vi "Compare and Append Cell.vi"(8 "Schedule Cell B in":refnum<class "Schedule Cell.lvclass">, 11 "Schedule Cell A in":refnum<class "Schedule Cell.lvclass">) -> (0 "Schedule Cell B out":refnum<class "Schedule Cell.lvclass">, 2 "Cell Updated":bool, 3 "Schedule Cell A out":refnum<class "Schedule Cell.lvclass">)   [LabVIEW 2020, in "Run Utilities.lvlib" / "Schedule Cell.lvclass"]
doc: "Compare two cells. If they have the same script the function modifies the cell A accordingly. Otherwise, the function returns unmodified cells."
uses:
  Schedule Cell.lvclass
  Schedule Cell.lvclass/Schedule Cell.ctl
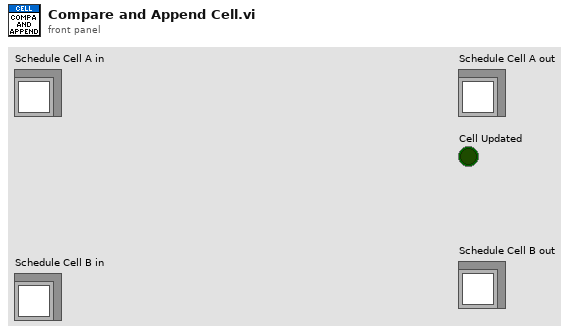
[diagram p1: front panel]
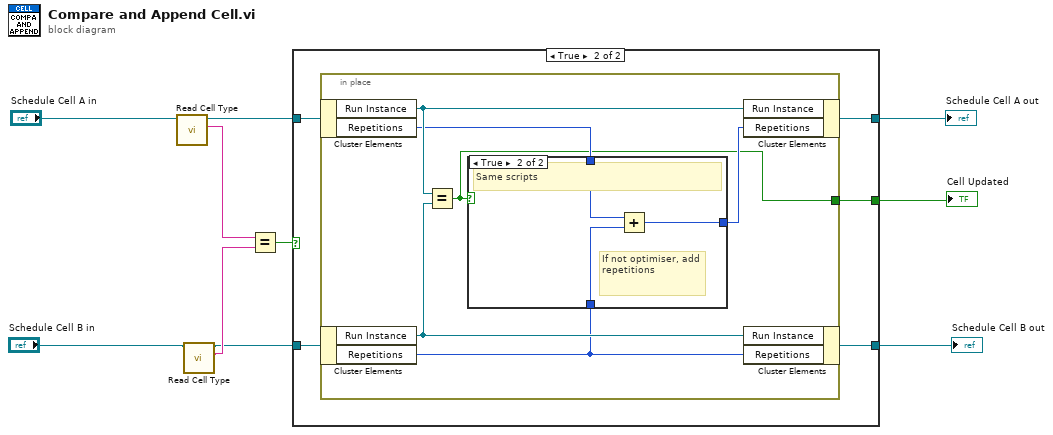
[diagram p0: block diagram]
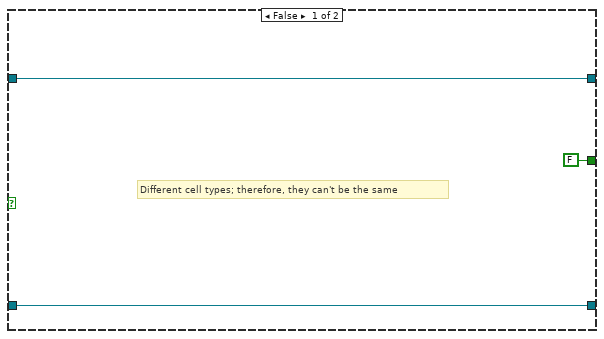
[diagram p2: hidden frame]
diagram:
  n1 = call-dynamic "Read Cell Type.vi"("Schedule Cell in"="Schedule Cell A in") -> ("Cell Type"=w3:string, "Schedule Cell out"=w4:refnum<class "Schedule Cell.lvclass">)  [unwired: 8 in, 1 out]
  n2 = call-dynamic "Read Cell Type.vi"("Schedule Cell in"="Schedule Cell B in") -> ("Cell Type"=w7:string, "Schedule Cell out"=w6:refnum<class "Schedule Cell.lvclass">)  [unwired: 8 in, 1 out]
  n3 = Equal?(x=w3, y=w7) -> (x = y?=w8:bool)
  n4 = case shown="True" w8 {
    tunnel: w4 -> [w12 w18]
    tunnel: [w12 w17] -> w1
    tunnel: [FALSE w16] -> w10
    tunnel: w6 -> [w13 w15]
    tunnel: [w13 w14] -> w9
    frame False {
      # "Different cell types; therefore, they can't be the same"
    }
    frame True {
      n5 = in-place {
        in-place-border: [w19] -> w16
        n6 = in-place-cluster #1(w18) -> ("Run Instance"=w23:refnum<class "Run Instance.lvclass">, "Repetitions"=w21:u32)
        n7 = in-place-cluster #2(w15) -> ("Run Instance"=w24:refnum<class "Run Instance.lvclass">, "Repetitions"=w22:u32)
        n8 = Equal?(x=w23, y=w24) -> (x = y?=w19:bool)
        n9 = case shown="True" w19 {
          tunnel: w22 -> [_ w28]
          tunnel: w21 -> [w25 w27]
          tunnel: [w25 w26] -> w20
          frame False {
            # "Different run cells, do nothing more"
          }
          frame True {
            # "If not optimiser, add repetitions"
            # "Same scripts"
            n10 = Add(x=w27, y=w28) -> (x+y=w26:u32)
          }
        }
        n11 = in-place-cluster #1("Run Instance"=w23, "Repetitions"=w20) -> (w17:refnum<class "Schedule Cell.lvclass">)
        n12 = in-place-cluster #2("Run Instance"=w24, "Repetitions"=w22) -> (w14:refnum<class "Schedule Cell.lvclass">)
      }
    }
  }
  "Schedule Cell A out" <- w1
  "Cell Updated" <- w10
  "Schedule Cell B out" <- w9
